vi "Configure Keyswitch.vi"(8 "error in (no error)":errorcluster, 9 "NIVS.System Definition Root":refnum<k24>, 10 "VI Reference":refnum<vi>, 11 "FNR Data in":T1) -> (0 "error out":errorcluster, 3 "FNR Data Out":T1)   [LabVIEW 2013]
doc: "Use this template to create a dialog box with event handling."
uses:
  NationalInstruments.VeriStand.SystemStorage
  Support/KeySwitch Parameters.ctl
  Support/PWM Object Parameters.ctl
  <vilib>/NI Veristand/UI Controls/Single Node Browser/NI_VS UI Single Node Browser.lvlib
  NationalInstruments.VeriStand.SystemStorageUI
panel:
  in  "Make Current Values Default":bool
  in  "Strings":string[](array[string])
  in  "PWM Array":dbl[](array[numeric]) min=0.0 max=1.0 step=0.0001
  in  "Keyswitch Positions":u8(knob)=2 scale=1.0..11.0
  in  "Lower Pane":u32(colorbox)=16777228
  in  "Upper Pane":u32(colorbox)=327424
  in  "RIO?":bool caption="Hardware type - click to toggle"
  in  "Control Label":string
  out "PWM Config Tab":enum32{"DAQ", "RIO"}(tab)
  in  "OK":bool
  in  "Cancel":bool
  in  "Selected Channel":refnum<k24>(container)
  # "Index (0-n)"
  # "There are transparent \ndecorations over the knob\nto prevent the user\nfrom changing the scale"
  # "PWM Duty Cycle"
  # "String Display"
  # "PWM"
  # "DAQ\nPWM\nRatio"
  # "FPGA\nPWM\n%"
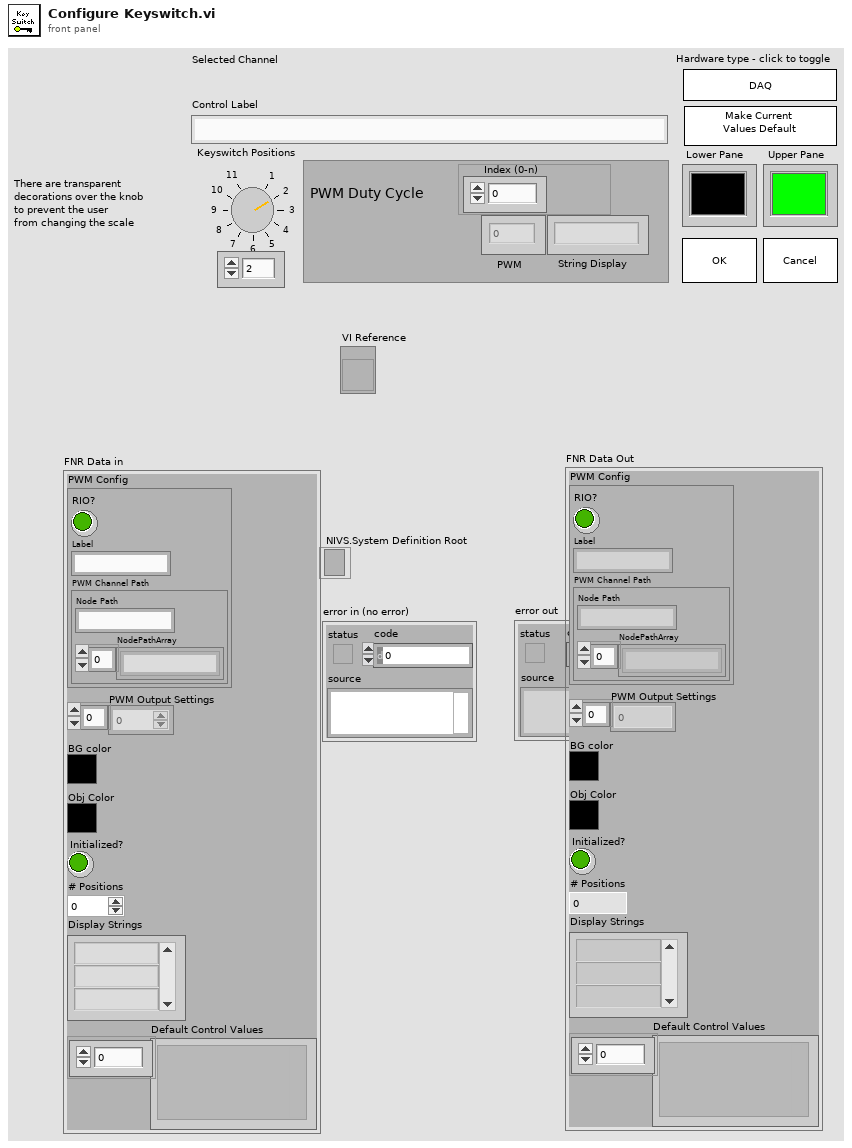
[diagram p1: front panel]
types:
  T1 = typedef "KeySwitch Parameters.ctl" = cluster{"PWM Config":T2, "PWM Output Settings":dbl[], "BG color":u32, "Obj Color":u32, "Initialized?":bool, "# Positions":u8, "Display Strings":string[], "Default Control Values":variant[]}
  T2 = typedef "PWM Object Parameters.ctl" = cluster{"RIO?":bool, "Label":string, "PWM Channel Path":cluster{"NodePathArray":string[], "Node Path":string}}
  T3 = typedef "NI_VS UI Single Node Browser.lvlib/Callback Type.ctl" = cluster{"Net Callbacks":refnum<k27>[], "Event":refnum<user-event>}
  T4 = typedef "NI_VS UI Single Node Browser.lvlib/Node Ref.ctl" = refnum<k24>
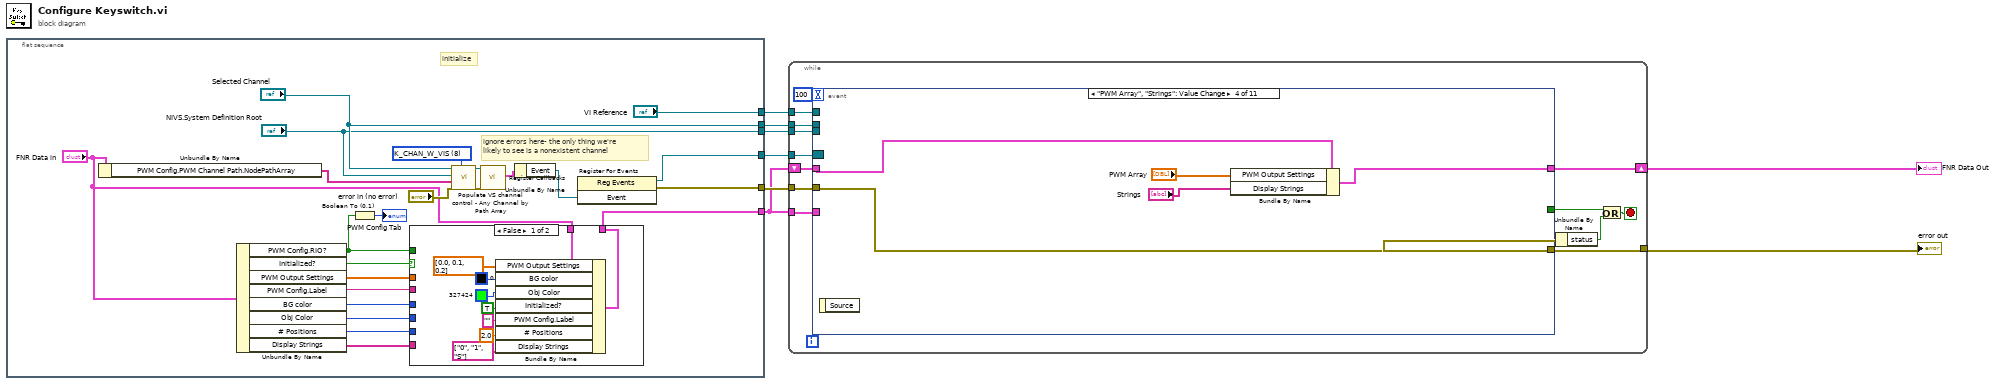
[diagram p0: block diagram]
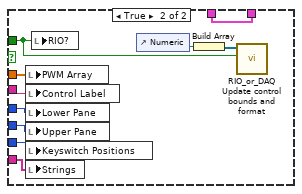
[diagram p2: hidden frame]
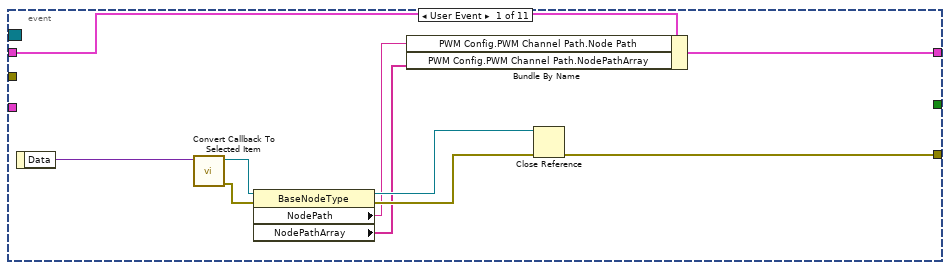
[diagram p3: hidden frame]
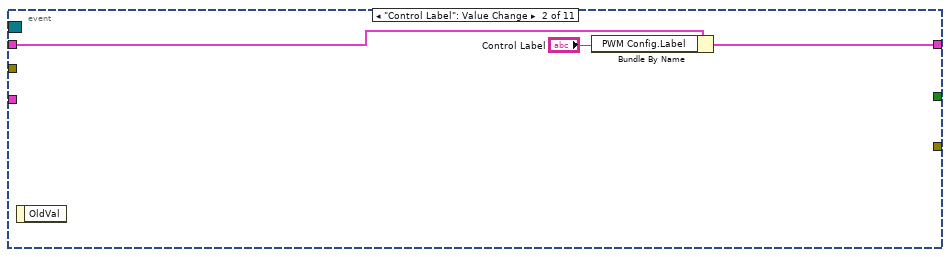
[diagram p4: hidden frame]
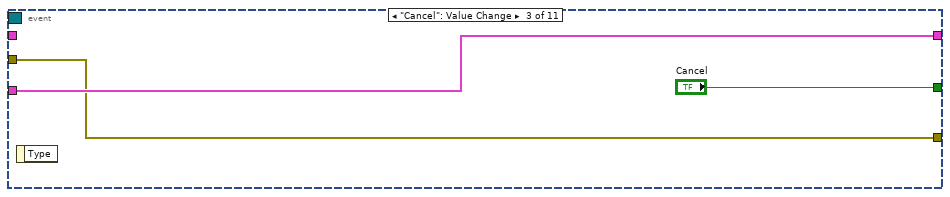
[diagram p5: hidden frame]
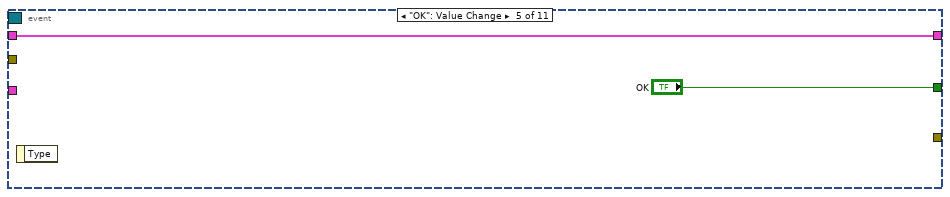
[diagram p6: hidden frame]
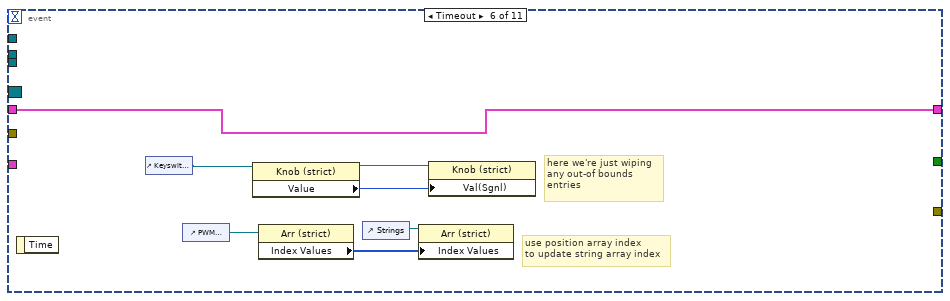
[diagram p7: hidden frame]
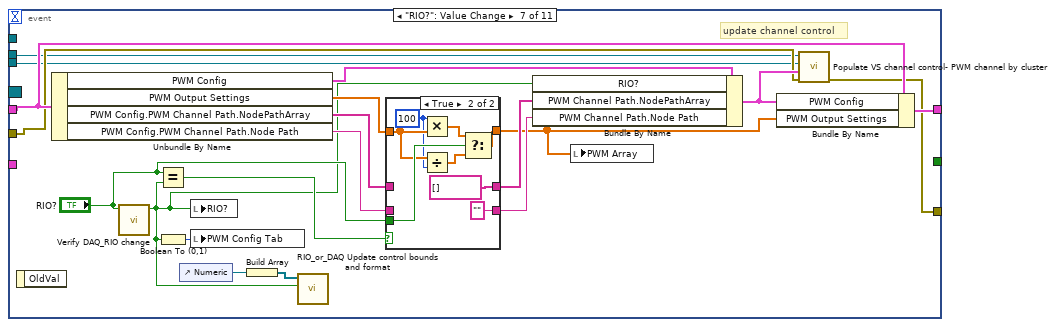
[diagram p8: hidden frame]
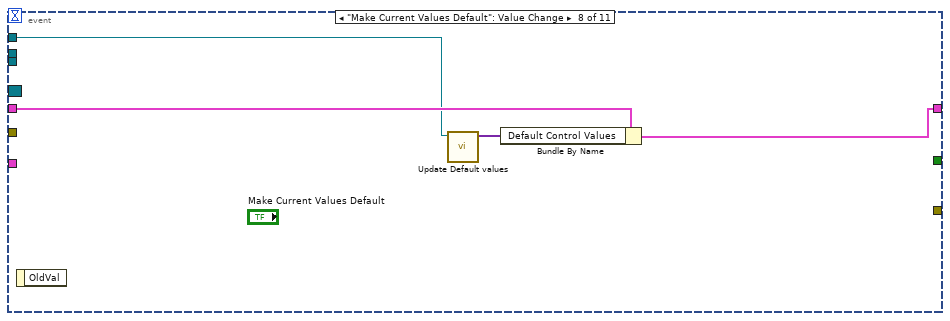
[diagram p10: hidden frame]
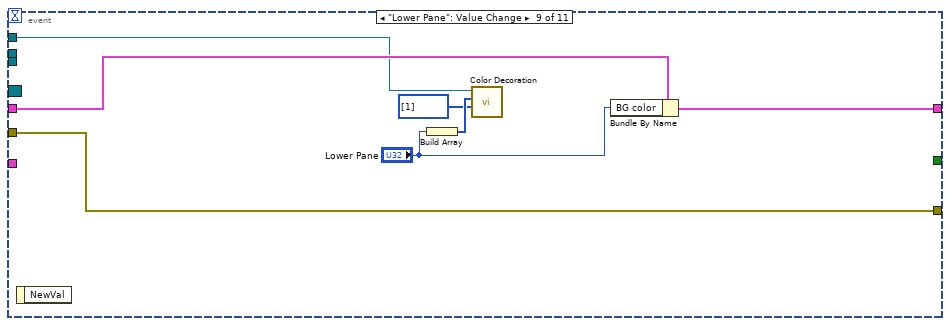
[diagram p11: hidden frame]
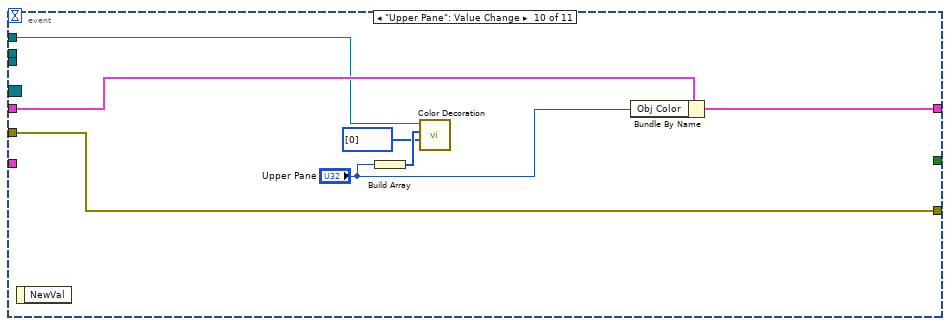
[diagram p12: hidden frame]
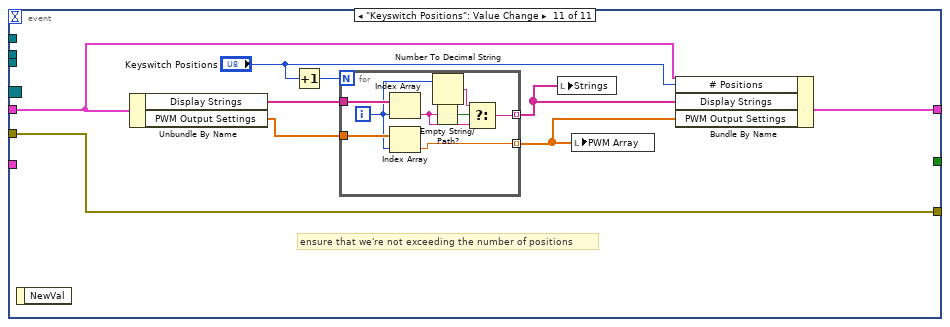
[diagram p13: hidden frame]
diagram:
  n1 = flat-sequence {
    tunnel: ["Selected Channel"] -> w7
    tunnel: ["NIVS.System Definition Root"] -> w6
    tunnel: [w15] -> w5
    tunnel: [w21] -> w1
    tunnel: ["VI Reference"] -> w3
    tunnel: [w14] -> w2
    frame #0 {
      w29 = u8 8 items=["K_CHAN_R", "K_CHAN_W", "K_CHAN_RW", "K_CHAN_VOLT", "K_CHAN_FAULT", "K_ALL", "K_CUSTOM", "K_CHAN_R_VIS", "K_CHAN_W_VIS", "K_CHAN_RW_VIS", "K_CHAN_VOLT_VIS", "K_CHAN_FAULT_VIS"] ("DisplayFilter")
      # "ignore errors here- the only thing we're\nlikely to see is a nonexistent channel"
      # "initialize"
      n2 = Unbundle By Name("FNR Data in") -> ("PWM Config.PWM Channel Path.NodePathArray"=w9:string[])
      n3 = Unbundle By Name("FNR Data in") -> ("PWM Config.RIO?"=w10:bool, "Initialized?"=w22:bool, "PWM Output Settings"=w26:dbl[], "PWM Config.Label"=w25:string, "BG color"=w24:u32, "Obj Color"=w23:u32, "# Positions"=w12:u8, "Display Strings"=w11:string[])
      n4 = Boolean To (0,1)(Boolean=w10) -> (0, 1=→"PWM Config Tab":i16)
      n5 = case shown="False" w22 {
        tunnel: w26 -> [_ w44]
        tunnel: w25 -> [_ w50]
        tunnel: w24 -> [_ w49]
        tunnel: w23 -> [_ w48]
        tunnel: "FNR Data in" -> [w40 w47]
        tunnel: [w39 w47] -> w21
        tunnel: w11 -> [_ w46]
        tunnel: w12 -> [_ w45]
        tunnel: w10 -> [_ w41]
        frame False {
          n6 = Bundle By Name(cluster=w40, "PWM Output Settings"=dbl[] [0.0, 0.1, 0.2] ("RIO PWM Settings"), "BG color"=u32 0, "Obj Color"=u32 327424, "Initialized?"=TRUE ("New?"), "PWM Config.Label"="" ("Label"), "# Positions"=2.0 ("# Pos"), "Display Strings"=string[] ["0", "1", "S"] ("Strings- DAQ")) -> (w39:T1)
        }
        frame True {
          n7 = local write "PWM Array"(w44) -> ()
          n8 = local write "Control Label"(w50) -> ()
          n9 = local write "Lower Pane"(w49) -> ()
          n10 = local write "Upper Pane"(w48) -> ()
          n11 = local write "Keyswitch Positions"(w45) -> ()
          n12 = local write "Strings"(w46) -> ()
          n13 = local write "RIO?"(w41) -> ()
          n14 = control-ref of="Numeric"() -> (w42:refnum<vi>)
          n15 = Build Array(w42) -> (w43:refnum<vi>[])
          n16 = call "RIO_or_DAQ Update control bounds and format.vi"("RIO? in"=w41, "Control References in"=w43) -> ()  [unwired: 10 in]
        }
      }
      n17 = call "Populate VS channel control - Any Channel by Path Array.vi"("DisplayFilter"=w29, "error in (no error)"="error in (no error)", "Path Array In"=w9, "NIVS.System Definition Root"="NIVS.System Definition Root", ".NET Refnum in"="Selected Channel") -> ("error out"=w16:errorcluster, ".NET Refnum out"=w17:refnum<k24>)  [unwired: 5 in]
      n18 = call <vilib>:"Register Callbacks.vi"("error in (no error)"=w16, "Single Node Browser"=w17) -> ("Callbacks"=w19:T3)  [unwired: 7 in, 2 out]
      n19 = Unbundle By Name(w19) -> ("Event"=w18:refnum<user-event>)
      n20 = register-events(w18) -> (reference out=w14:refnum<event-registration>, error out=w15:errorcluster)  [unwired: 2 in]
    }
  }
  n21 = while {
    tunnel: [w62] -> w8
    shift-right: [w58] -> w4
    shift-left: w1 -> [w60]
    tunnel: w1 -> [w59]
    tunnel: w7 -> [w56]
    tunnel: w6 -> [w55]
    tunnel: w5 -> [w54]
    tunnel: w3 -> [w53]
    tunnel: w2 -> [w52]
    stop <- w57 stop-if-true
    n22 = event shown="[3] \"PWM Array\", \"Strings\": Value Change" {
      selector: w52 -> [_ _ _ _ _ _ _ _ _ _ _]
      dyn-events: _ -> [_ _ _ _ _ _ _ _ _ _ _]
      timeout: 100 -> [_ _ _ _ _ _ _ _ _ _ _]
      tunnel: [_ _ "Cancel" _ "OK" _ _ _ _ _ _] -> w63
      tunnel: [w66 _ w77 w84 _ _ w96 _ w133 w140 w151] -> w62
      tunnel: w60 -> [w67 w75 _ w80 w85 w90 w105 w127 w134 w141 w150]
      tunnel: w59 -> [_ _ w78 _ _ _ _ _ _ _ _]
      tunnel: [w65 w76 w78 w83 w85 w90 w97 w125 w135 w142 w149] -> w58
      tunnel: w56 -> [_ _ _ _ _ _ w103 _ _ _ _]
      tunnel: w55 -> [_ _ _ _ _ _ w102 _ _ _ _]
      tunnel: w54 -> [_ _ w77 w84 _ _ w104 _ w133 w140 w151]
      tunnel: w53 -> [_ _ _ _ _ _ _ w126 w129 w136 _]
      event User Event {
        n23 = event-data() -> ("Data"=w68:variant)  [unwired: 1 in]
        n24 = call <vilib>:"Convert Callback To Selected Item.vi"("Data"=w68) -> ("error out"=w70:errorcluster, "Selected Item"=w73:T4)  [unwired: 9 in]
        n25 = property class="BaseNodeType"(reference=w73, error in=w70) -> (reference out=w72:T4, error out=w71:errorcluster, "NodePath"=w64:string, "NodePathArray"=w69:string[])
        n26 = Bundle By Name(cluster=w67, "PWM Config.PWM Channel Path.Node Path"=w64, "PWM Config.PWM Channel Path.NodePathArray"=w69) -> (w65:T1)
        n27 = Close Reference(reference=w72, error in (no error)=w71) -> (error out=w66:errorcluster)
      }
      event "Control Label": Value Change {
        n28 = event-data() -> ()  [unwired: 1 in, 1 out]
        n29 = Bundle By Name(cluster=w75, "PWM Config.Label"="Control Label") -> (w76:T1)
      }
      event "Cancel": Value Change {
        n30 = event-data() -> ()  [unwired: 1 in, 1 out]
      }
      event "PWM Array", "Strings": Value Change {
        n31 = event-data() -> ()  [unwired: 1 in, 1 out]
        n32 = Bundle By Name(cluster=w80, "PWM Output Settings"="PWM Array", "Display Strings"="Strings") -> (w83:T1)
      }
      event "OK": Value Change {
        n33 = event-data() -> ()  [unwired: 1 in, 1 out]
      }
      event Timeout {
        # "use position array index \nto update string array index"
        # "here we're just wiping\nany out-of bounds\nentries"
        n34 = event-data() -> ()  [unwired: 1 in, 1 out]
        n35 = control-ref of="Keyswitch Positions"() -> (w87:refnum<vi>)
        n36 = control-ref of="PWM Array"() -> (w92:refnum<vi>)
        n37 = property class="Knob (strict)"(reference=w87) -> (reference out=w88:refnum<vi>, "Value"=w89:u8)  [unwired: 1 in, 1 out]
        n38 = property class="Arr (strict)"(reference=w92) -> ("Index Values"=w93:u32[])  [unwired: 1 in, 2 out]
        n39 = control-ref of="Strings"() -> (w91:refnum<vi>)
        n40 = property class="Arr (strict)"(reference=w91, "Index Values"=w93) -> ()  [unwired: 1 in, 2 out]
        n41 = property class="Knob (strict)"(reference=w88, "Val(Sgnl)"=w89) -> ()  [unwired: 1 in, 2 out]
      }
      event "RIO?": Value Change {
        # "update channel control"
        n42 = event-data() -> ()  [unwired: 1 in, 1 out]
        n43 = Unbundle By Name(w105) -> ("PWM Config"=w113:T2, "PWM Output Settings"=w111:dbl[], "PWM Config.PWM Channel Path.NodePathArray"=w110:string[], "PWM Config.PWM Channel Path.Node Path"=w109:string)
        n44 = call "Verify DAQ_RIO change.vi"("RIO? in"="RIO?") -> ("RIO? out"=w100:bool)  [unwired: 10 in]
        n45 = Equal?(x="RIO?", y=w100) -> (x = y?=w108:bool)
        n46 = Boolean To (0,1)(Boolean=w100) -> (0, 1=w99:i16)
        n47 = control-ref of="Numeric"() -> (w95:refnum<vi>)
        n48 = local write "RIO?"(w100) -> ()
        n49 = local write "PWM Config Tab"(w99) -> ()
        n50 = Build Array(w95) -> (w94:refnum<vi>[])
        n51 = call "RIO_or_DAQ Update control bounds and format.vi"("RIO? in"=w100, "Control References in"=w94) -> ()  [unwired: 10 in]
        n52 = case shown="True" w108 {
          tunnel: w111 -> [w116 w119]
          tunnel: "RIO?" -> [_ w123]
          tunnel: [w116 w122] -> w98
          tunnel: w110 -> [w115 _]
          tunnel: [w115 string[] [] ("NodePathArray")] -> w107
          tunnel: w109 -> [w114 _]
          tunnel: [w114 "" ("Node Path")] -> w106
          frame False {
          }
          frame True {
            w118 = 100
            n53 = Multiply(x=w118, y=w119) -> (x*y=w124:dbl[])
            n54 = Divide(x=w119, y=w118) -> (x/y=w121:dbl[])
            n55 = Select(t=w124, s=w123, f=w121) -> (s? t:f=w122:dbl[])
          }
        }
        n56 = Bundle By Name(cluster=w113, "RIO?"=w100, "PWM Channel Path.NodePathArray"=w107, "PWM Channel Path.Node Path"=w106) -> (w112:T2)
        n57 = local write "PWM Array"(w98) -> ()
        n58 = Bundle By Name(cluster=w105, "PWM Config"=w112, "PWM Output Settings"=w98) -> (w97:T1)
        n59 = call "Populate VS channel control- PWM channel by cluster.vi"("error in (no error)"=w104, "Data cluster in"=w112, "NIVS.System Definition Root"=w102, ".NET Refnum in"=w103) -> ("error out"=w96:errorcluster)  [unwired: 6 in, 1 out]
      }
      event "Make Current Values Default": Value Change {
        n60 = event-data() -> ()  [unwired: 1 in, 1 out]
        n61 = call "Update Default values.vi"("VI in"=w126) -> ("Default Values out"=w128:variant[])  [unwired: 10 in]
        n62 = Bundle By Name(cluster=w127, "Default Control Values"=w128) -> (w125:T1)
      }
      event "Lower Pane": Value Change {
        n63 = event-data() -> ()  [unwired: 1 in, 1 out]
        n64 = Build Array("Lower Pane") -> (w132:u32[])
        n65 = call "Color Decoration.vi"("VI reference"=w129, "Color Array"=w132, "Index Array"=u32[] [1]) -> ()  [unwired: 7 in, 1 out]
        n66 = Bundle By Name(cluster=w134, "BG color"="Lower Pane") -> (w135:T1)
      }
      event "Upper Pane": Value Change {
        n67 = event-data() -> ()  [unwired: 1 in, 1 out]
        n68 = Build Array("Upper Pane") -> (w139:u32[])
        n69 = call "Color Decoration.vi"("VI reference"=w136, "Color Array"=w139, "Index Array"=u32[] [0]) -> ()  [unwired: 7 in, 1 out]
        n70 = Bundle By Name(cluster=w141, "Obj Color"="Upper Pane") -> (w142:T1)
      }
      event "Keyswitch Positions": Value Change {
        # "ensure that we're not exceeding the number of positions"
        n71 = event-data() -> ()  [unwired: 1 in, 1 out]
        n72 = Unbundle By Name(w150) -> ("Display Strings"=w147:string[], "PWM Output Settings"=w145:dbl[])
        n73 = Increment(x="Keyswitch Positions") -> (x+1=w148:u8)
        n74 = for {
          N: w148 -> [_]
          tunnel: [w158] -> w144 mode=indexing
          tunnel: w147 -> [w157]
          tunnel: w145 -> [w156]
          tunnel: [w153] -> w143 mode=indexing
          i -> [w152]
          n75 = Index Array(array=w157, index=w152) -> (element=w154:string)
          n76 = Index Array(array=w156, index=w152) -> (element=w153:dbl)
          n77 = Empty String/Path?(string/path=w154) -> (empty?=w159:bool)
          n78 = Number To Decimal String(number=w152) -> (decimal integer string=w155:string)  [unwired: 1 in]
          n79 = Select(t=w155, s=w159, f=w154) -> (s? t:f=w158:string)
        }
        n80 = local write "Strings"(w144) -> ()
        n81 = local write "PWM Array"(w143) -> ()
        n82 = Bundle By Name(cluster=w150, "# Positions"="Keyswitch Positions", "Display Strings"=w144, "PWM Output Settings"=w143) -> (w149:T1)
      }
    }
    n83 = Unbundle By Name(w62) -> ("status"=w61:bool)
    n84 = Or(x=w63, y=w61) -> (x .or. y?=w57:bool)
  }
  "error out" <- w8
  "FNR Data Out" <- w4
